vi "Calc phase increase and offset.vi"(6 "Phase offset":dbl, 7 "# of DDS":i32=4, 8 "error in (no error)":errorcluster, 9 "resolution (32bit)":i32=32, 10 "fclk (800MHz)":dbl=800000000.0 format="%#_6p", 11 "f_generated (MHz)":dbl=10.0) -> (0 "error out":errorcluster, 2 "Phase out":fxp<+,64,64>[](array[numeric]), 3 "delta":dbl)   [LabVIEW 2013]
doc: "Calculates Phase Increment (\"pinc\") information for DDS core."
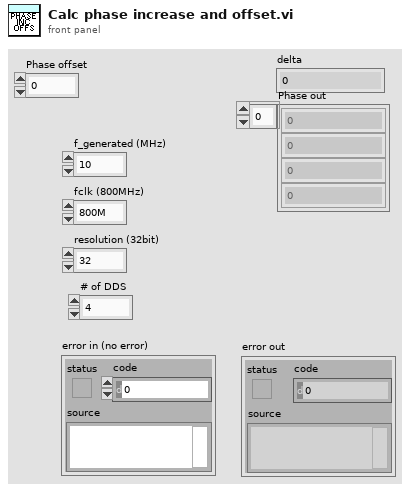
[diagram p1: front panel]
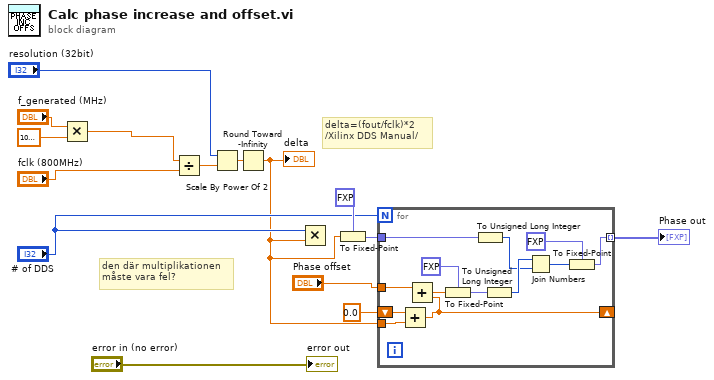
[diagram p0: block diagram]
diagram:
  # "den där multiplikationen\nmåste vara fel?"
  # "delta=(fout/fclk)*2\n/Xilinx DDS Manual/"
  n1 = Multiply(x="f_generated (MHz)", y=1000000.0) -> (x*y=w3:dbl)
  n2 = Divide(x=w3, y="fclk (800MHz)") -> (x/y=w14:dbl)
  n3 = Scale By Power Of 2(n="resolution (32bit)", x=w14) -> (x*2^n=w10:dbl)
  n4 = Round Toward -Infinity(1:w10) -> (0:w1:dbl)
  "delta" <- w1
  n5 = Multiply(x="# of DDS", y=w1) -> ()  [unwired: 1 out]
  n6 = To Fixed-Point(fixed-point type=fxp<+,32,32> 0.0 ("pinc_in0"), number=w1) -> (fixed-point=w11:fxp<+,32,32>)
  n7 = for {
    N: "# of DDS" -> [_]
    tunnel: w11 -> [w22]
    tunnel: [w16] -> w5 mode=indexing
    tunnel: w1 -> [w28]
    shift-right: [w25] -> _
    shift-left: 0.0 -> [w26]
    tunnel: "Phase offset" -> [w24]
    n8 = Add(x=w26, y=w28) -> (x+y=w25:dbl)
    n9 = Add(x=w24, y=w25) -> (x+y=w23:dbl)
    n10 = To Fixed-Point(fixed-point type=fxp<+,32,32> 0.0 ("pinc_in0"), number=w23) -> (fixed-point=w21:fxp<+,32,32>)
    n11 = To Unsigned Long Integer(number=w22) -> (unsigned 32bit integer=w19:u32)
    n12 = To Unsigned Long Integer(number=w21) -> (unsigned 32bit integer=w20:u32)
    n13 = Join Numbers(hi=w20, lo=w19) -> ((hi.lo)=w18:u64)
    n14 = To Fixed-Point(fixed-point type=fxp<+,64,64> 0.0, number=w18) -> (fixed-point=w16:fxp<+,64,64>)
  }
  "Phase out" <- w5
  "error out" <- "error in (no error)"
